vi "STFT Spectrogram.vi"(2 "window selector":i32(ring) items=["Rectangular", "Blackman", "Hamming", "Hanning", "Gaussian"], 3 "window length":i32=4 min=0, 4 "time increment":i32=1 min=0, 5 "X":dbl[](array[numeric])) -> (0 "error":i32, 1 "STFT Spectrogram {X}":dbl[][](array[numeric]))   [LabVIEW 2014, in "NI_Gmath.lvlib"]
doc: "Computes the signal energy distribution in the joint time-frequency domain, using the Short-Time Fourier Transform (STFT) algorithm."
uses:
  NI_Gmath.lvlib
  Blackman Window (DBL).vi
  Hamming Window (DBL).vi
  Hanning Window (DBL).vi
  Unit Vector (DBL).vi
  AllCosWindow (DBL).vi
  NI_AALPro.lvlib
  NI_AALBase.lvlib
panel:
  # "This VI is obsolete !!!\nYou should replace this VI in your diagram with the STFT Spectrograms VI.  \n\nNOTE: If you have wired to the window selector input of this obsolete VI, please be aware that the window selector input in STFT Spectrograms VI is different."
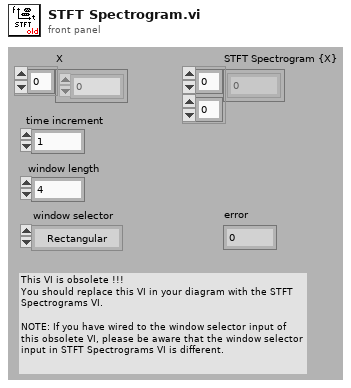
[diagram p1: front panel]
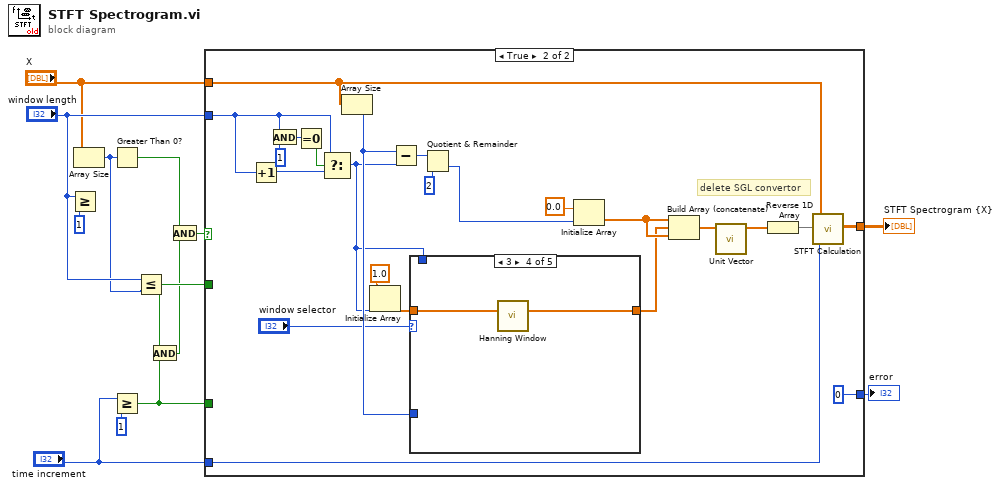
[diagram p0: block diagram]
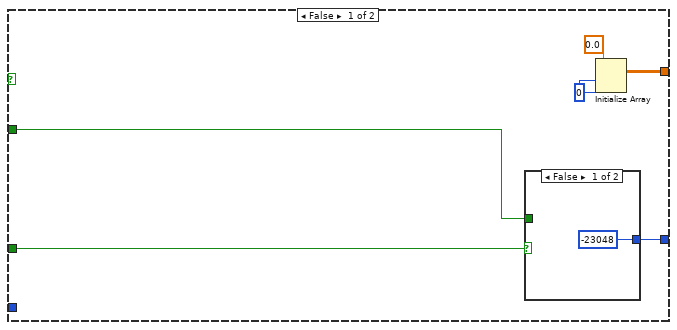
[diagram p2: hidden frame]
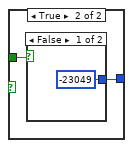
[diagram p3: hidden frame]
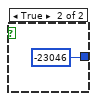
[diagram p4: hidden frame]
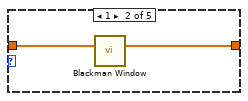
[diagram p6: hidden frame]
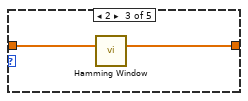
[diagram p7: hidden frame]
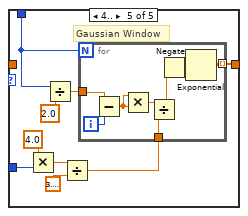
[diagram p8: hidden frame]
diagram:
  n1 = Greater Or Equal?(x="window length", y=1) -> ()  [unwired: 1 out]
  n2 = Array Size(array="X") -> (size(s)=w7:i32)
  n3 = Greater Than 0?(x=w7) -> (x > 0?=w5:bool)
  n4 = Greater Or Equal?(x="time increment", y=1) -> (x >= y?=w2:bool)
  n5 = Less Or Equal?(x="window length", y=w7) -> (x <= y?=w6:bool)
  n6 = And(x=w6, y=w2) -> (x .and. y?=w4:bool)
  n7 = And(x=w5, y=w4) -> (x .and. y?=w3:bool)
  n8 = case shown="True" w3 {
    tunnel: [w17 w47] -> w13
    tunnel: "X" -> [_ w45]
    tunnel: "window length" -> [_ w34]
    tunnel: [w15 0] -> w12
    tunnel: "time increment" -> [_ w26]
    tunnel: w2 -> [w16 _]
    tunnel: w6 -> [w14 _]
    frame False {
      w18 = 0
      n9 = case shown="False" w16 {
        tunnel: [-23048 w21] -> w15
        tunnel: w14 -> [_ w22]
        frame False {
        }
        frame True {
          n10 = case shown="False" w22 {
            tunnel: [-23049 -23046] -> w21
            frame False {
            }
            frame True {
            }
          }
        }
      }
      n11 = Initialize Array(sgl 0.0, w18, w18) -> (w17:sgl[][])
    }
    frame True {
      # "delete SGL convertor"
      n12 = Increment(x=w34) -> (x+1=w32:i32)
      n13 = And(x=w34, y=1) -> (x .and. y?=w30:i32)
      n14 = Equal To 0?(x=w30) -> (x = 0?=w31:bool)
      n15 = Select(t=w34, s=w31, f=w32) -> (s? t:f=w39:i32)
      n16 = Array Size(array=w45) -> (size(s)=w44:i32)
      n17 = Initialize Array(1.0, w39) -> (w38:dbl[])
      n18 = Subtract(x=w44, y=w39) -> (x-y=w42:i32)
      n19 = case shown="3" "window selector" {
        tunnel: w44 -> [_ _ _ _ w57]
        tunnel: [w48 w49 w51 w53 w60] -> w33
        tunnel: w38 -> [w48 w50 w52 w54 _]
        tunnel: w39 -> [_ _ _ _ w59]
        frame ..0 {
          # "Rectangular"
        }
        frame 1 {
          n20 = call-poly "Blackman Window.vi"("X"=w50) -> ("Windowed X"=w49:dbl[])  [unwired: 1 out]
        }
        frame 2 {
          n21 = call-poly "Hamming Window.vi"("X"=w52) -> ("Windowed X"=w51:dbl[])  [unwired: 1 out]
        }
        frame 3 {
          n22 = call-poly "Hanning Window.vi"("X"=w54) -> ("Windowed X"=w53:dbl[])  [unwired: 1 out]
        }
        frame 4.. {
          # "Gaussian Window"
          n23 = Multiply(x=4.0, y=w57) -> (x*y=w58:dbl)
          n24 = Divide(x=w59, y=2.0) -> (x/y=w62:dbl)
          n25 = Divide(x=w58, y=3.141592653589793) -> (x/y=w61:dbl)
          n26 = for {
            N: w59 -> [_]
            tunnel: [w66] -> w60 mode=indexing
            tunnel: w61 -> [w69]
            tunnel: w62 -> [w64]
            i -> [w71]
            n27 = Subtract(x=w64, y=w71) -> (x-y=w65:dbl)
            n28 = Multiply(x=w65, y=w65) -> (x*y=w70:dbl)
            n29 = Divide(x=w70, y=w69) -> (x/y=w68:dbl)
            n30 = Negate(x=w68) -> (-x=w67:dbl)
            n31 = Exponential(1:w67) -> (0:w66:dbl)
          }
        }
      }
      n32 = Quotient & Remainder(x=w42, y=2) -> (floor(x/y)=w41:i32)  [unwired: 1 out]
      n33 = Initialize Array(0.0, w41) -> (w36:dbl[])
      n34 = Build Array (concatenate)(w36, w33, w36) -> (w40:dbl[])
      n35 = call-poly "Unit Vector.vi"("Input Vector"=w40) -> ("Unit Vector"=w25:dbl[])  [unwired: 8 in, 2 out]
      n36 = Reverse 1D Array(array=w25) -> (reversed array=w46:dbl[])
      n37 = call "STFT Calculation.vi"("time increment"=w26, "g"=w46, "s"=w45) -> ("Fourier[s(i-m)*g(m)]"=w47:dbl[][])
    }
  }
  "STFT Spectrogram {X}" <- w13
  "error" <- w12
